vi "ModbusVi2.vi"(7 "VISA resource name":refnum<visa-resource-name>, 8 "error in":errorcluster, 9 "Holding Register":u16, 10 "Scalling":dbl, 11 "Offset":dbl) -> (0 "error out":errorcluster, 1 "error de conexion":bool, 2 "Value":dbl, 3 "Value Register":u16[](array[numeric]))   [LabVIEW 2015]
uses:
  <vilib>/NI/Modbus Library/API/Master/Modbus Master.lvclass
  <vilib>/NI/Modbus Library/API/Wrapper/Create Serial Master.vi
panel:
  # "LECTURA DE VOLTAJE DE BATERIA"
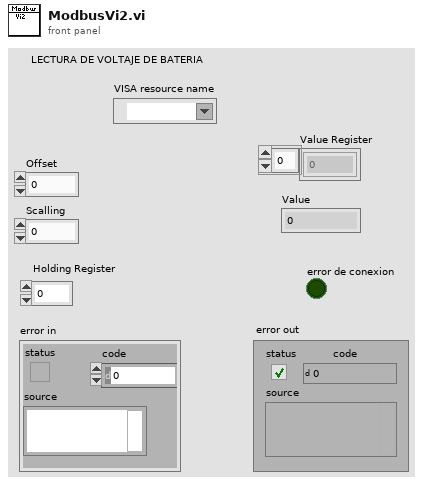
[diagram p1: front panel]
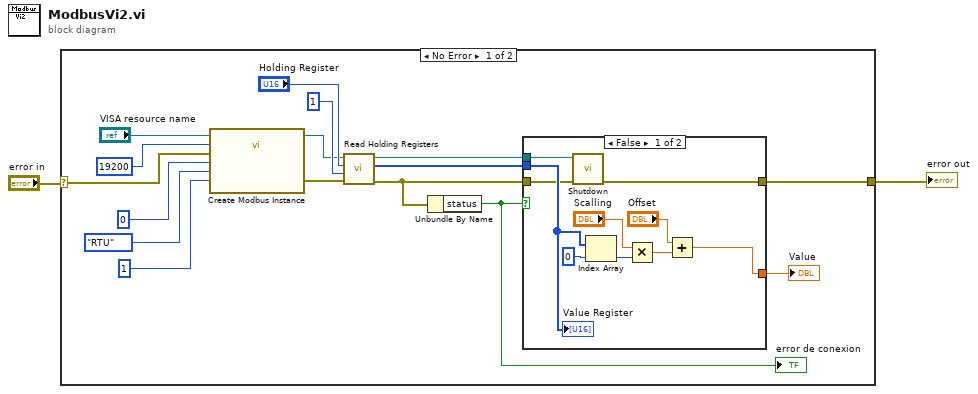
[diagram p0: block diagram]
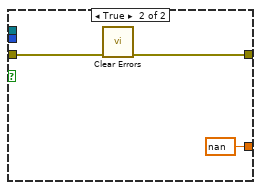
[diagram p2: hidden frame]
diagram:
  n1 = case shown="No Error" "error in" {
    selector: "error in" -> [w4 w32]
    tunnel: [w3 w32] -> w1
    frame No Error {
      n2 = call-poly <vilib>:"Create Modbus Instance.vi"("serial type"=enum16{"RTU", "ASCII"}."RTU", "parity (even)"=0, "unit ID"=u8 1, "error in"=w4, "baud rate"=u32 19200, "VISA resource name"="VISA resource name") -> ("error out"=w8:errorcluster, "serial master instance"=w14:refnum<class "Modbus Master.lvclass">)  [unwired: 4 in]
      n3 = call-dynamic "Read Holding Registers.vi"("error in"=w8, "number of inputs"=1, "starting address"="Holding Register", "Modbus master in"=w14) -> ("error out"=w6:errorcluster, "register values"=w16:u16[], "Modbus master out"=w15:refnum<class "Modbus Master.lvclass">)  [unwired: 5 in]
      n4 = Unbundle By Name(w6) -> ("status"=w5:bool)
      "error de conexion" <- w5
      n5 = case shown="False" w5 {
        tunnel: w16 -> [w26 _]
        tunnel: w15 -> [w24 _]
        tunnel: [w21 nan] -> w7
        tunnel: [w20 w29] -> w3
        tunnel: w6 -> [w19 w30]
        frame False {
          n6 = call-dynamic "Shutdown.vi"("error in"=w19, "Modbus master in"=w24) -> ("error out"=w20:errorcluster)  [unwired: 9 in]
          n7 = Index Array(array=w26, index=0) -> (element=w27:u16)
          n8 = Multiply(x="Scalling", y=w27) -> (x*y=w22:dbl)
          n9 = Add(x="Offset", y=w22) -> (x+y=w21:dbl)
          "Value Register" <- w26
        }
        frame True {
          n10 = call <vilib>:"Clear Errors.vi"("error in (no error)"=w30) -> ("error out"=w29:errorcluster)  [unwired: 5 in, 1 out]
        }
      }
      "Value" <- w7
    }
    frame Error {
    }
  }
  "error out" <- w1
